vi "Sound Warning.vi"(8 "error in (no error)":errorcluster, 11 "Electric Fences in":refnum<class "Electric Fences.lvclass">) -> (0 "error out":errorcluster, 3 "Electric Fences out":refnum<class "Electric Fences.lvclass">)   [LabVIEW 2020, in "Electric Fences.lvclass"]
uses:
  Electric Fences.lvclass
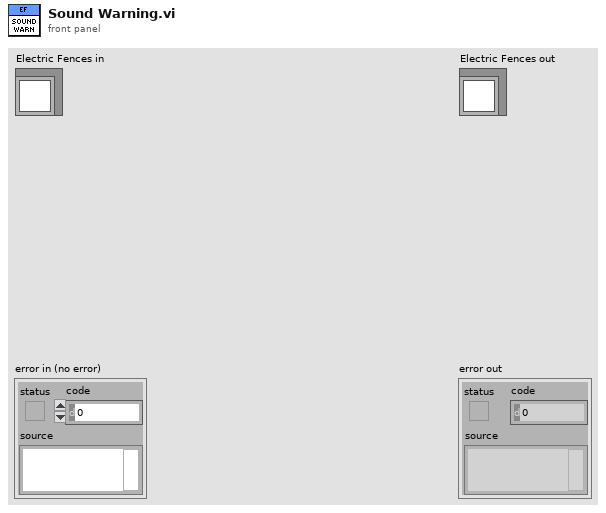
[diagram p1: front panel]
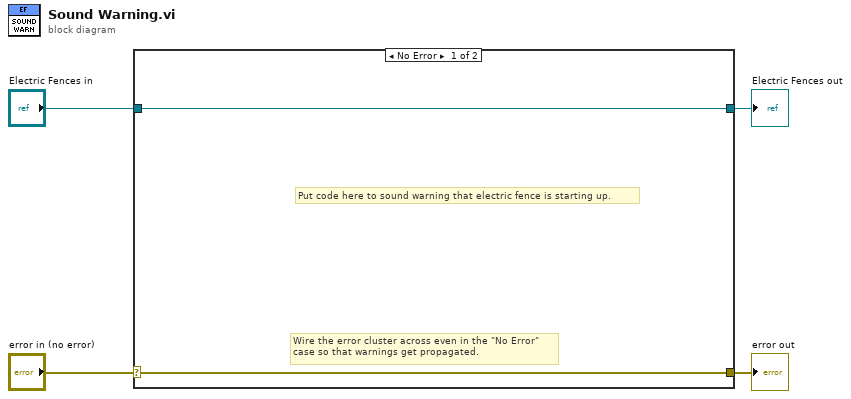
[diagram p0: block diagram]
diagram:
  n1 = case shown="No Error" "error in (no error)" {
    selector: "error in (no error)" -> [w5 w8]
    tunnel: [w5 w8] -> w3
    tunnel: [w6 w7] -> w1
    tunnel: "Electric Fences in" -> [w6 w7]
    frame No Error {
      # "Put code here to sound warning that electric fence is starting up."
      # "Wire the error cluster across even in the \"No Error\"\ncase so that warnings get propagated."
    }
    frame Error {
    }
  }
  "error out" <- w3
  "Electric Fences out" <- w1
